vi "FTW-ActorExtended-Child-Add.vi"(0 "FTW-ActorExtended In":refnum<class "FTW-ActorExtended.lvclass">, 5 "Identity":string, 7 "Inbox Address":string, 9 "Connection":refnum<class "FTW-ActorConnector.lvclass">, 11 "error in":errorcluster) -> (4 "FTW-ActorExtended Out":refnum<class "FTW-ActorExtended.lvclass">, 15 "error out":errorcluster)   [LabVIEW 2013, in "FTW-ActorExtended.lvclass"]
uses:
  FTW-ActorExtended.lvclass
  Connector/FTW-ActorConnector.lvclass
  FTW-ActorExtended.lvclass/FTW-ActorExtended.ctl
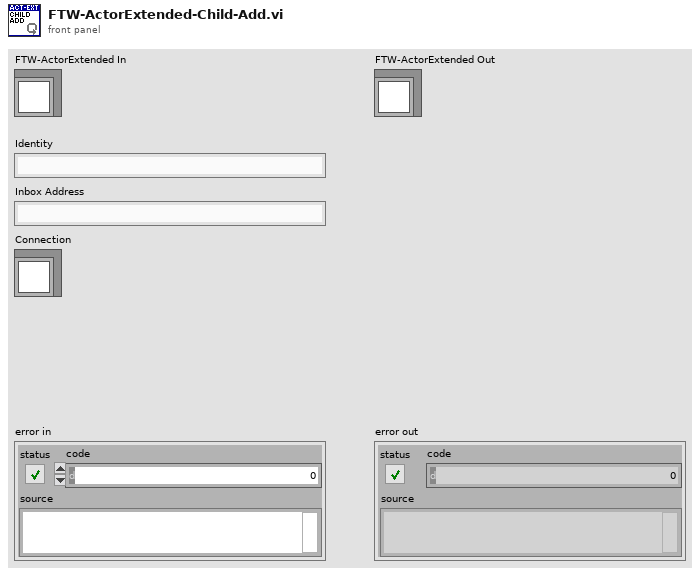
[diagram p1: front panel]
types:
  T1 = cluster{"Identity":string, "Inbox Address":string, "Connection":refnum<class "FTW-ActorConnector.lvclass">}
  T2 = cluster{"Name":string, "URI":string, "Connector":refnum<class "FTW-ActorConnector.lvclass">}[]
  T3 = cluster{"Identity":string, "Inbox Address":string, "Connection":refnum<class "FTW-ActorConnector.lvclass">}[]
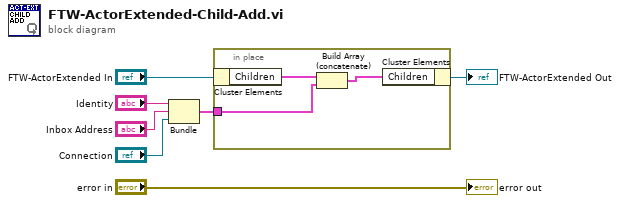
[diagram p0: block diagram]
diagram:
  n1 = Bundle("Identity"="Identity", "Inbox Address"="Inbox Address", "Connection"="Connection") -> (w3:T1)  [unwired: 1 in]
  n2 = in-place {
    in-place-border: w3 -> [w8]
    n3 = in-place-cluster #1("FTW-ActorExtended In") -> ("Children"=w10:T2)
    n4 = Build Array (concatenate)(w10, w8) -> (w9:T3)
    n5 = in-place-cluster #1("Children"=w9) -> (→"FTW-ActorExtended Out":refnum<class "FTW-ActorExtended.lvclass">)
  }
  "error out" <- "error in"
